vi "Get median.vi"(7 "N":i32=20, 11 "DataIn":i16) -> (1 "Median":i16, 2 "Ready":bool, 3 "ArrayOut":i16[](array[numeric]))   [LabVIEW 2015]
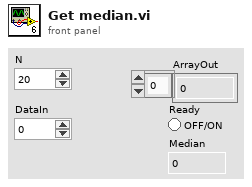
[diagram p1: front panel]
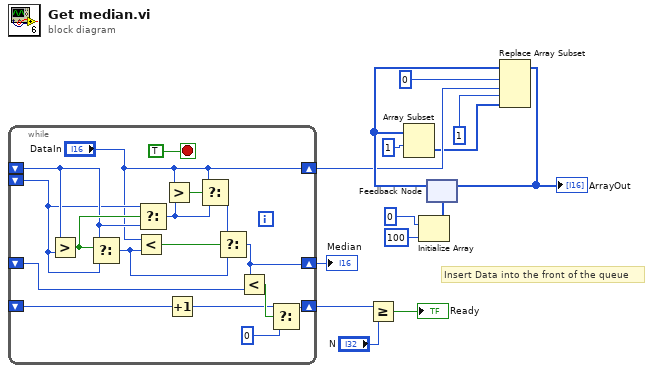
[diagram p0: block diagram]
diagram:
  # "Insert Data into the front of the queue"
  n1 = while {
    shift-right: ["DataIn"] -> w4
    shift-left: _ -> [w25]
    shift-left: _ -> [w24]
    shift-right: [w28] -> w14
    shift-left: _ -> [w27]
    shift-right: [w18] -> w8
    shift-left: _ -> [w17]
    stop <- TRUE stop-if-true
    n2 = Greater?(x=w25, y=w24) -> (0:w26:bool)
    n3 = Select(t=w25, s=w26, f=w24) -> (s? t:f=w29:i16)
    n4 = Less?(x="DataIn", y=w29) -> (x < y?=w30:bool)
    n5 = Select(t=w24, s=w26, f=w25) -> (s? t:f=w22:i16)
    n6 = Greater?(x="DataIn", y=w22) -> (0:w23:bool)
    n7 = Increment(x=w17) -> (x+1=w16:i32)
    n8 = Select(t="DataIn", s=w23, f=w22) -> (s? t:f=w21:i16)
    n9 = Select(t=w21, s=w30, f=w29) -> (s? t:f=w28:i16)
    n10 = Less?(x=w28, y=w27) -> (x < y?=w20:bool)
    n11 = Select(t=w16, s=w20, f=0 ("Address")) -> (s? t:f=w18:i32)
  }
  "Median" <- w14
  n12 = Greater Or Equal?(x=w8, y="N") -> (x >= y?=→"Ready":bool)
  n13 = Initialize Array(i16 0 ("DataIn"), 100 ("dimension size")) -> (w10:i16[])
  n14 = feedback #1(w10) -> (w6:i16[])
  n15 = Array Subset(array=w6, index=1) -> (w2:i16[])  [unwired: 1 in]
  n16 = Replace Array Subset(array=w6, new element #1=w4, index #1=0 ("index"), new element #2=w2, index #2=1 ("index")) -> (w1:i16[])
  "ArrayOut" <- w1
  n17 = feedback-in #1(w1) -> ()
